vi "mclamp_set_holding.vi"(8 "error in (no error)":errorcluster, 9 "set holding (mV)":dbl, 10 "Error in":i32, 11 "Multiclamp Handle Out":u32) -> (0 "error out":errorcluster, 2 "error out":i32)   [LabVIEW 2015]
uses:
  multiBot/patcherBot/AxMultiClampMsg.dll
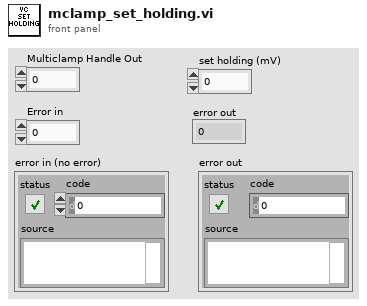
[diagram p1: front panel]
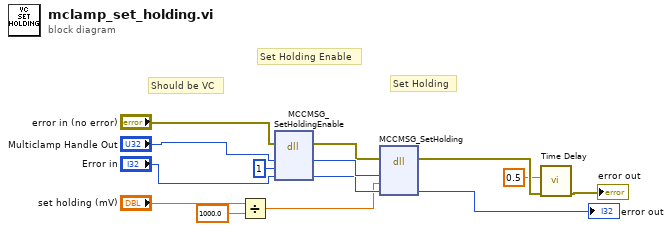
[diagram p0: block diagram]
diagram:
  # "Set Holding Enable"
  # "Set Holding"
  # "Should be VC"
  n1 = Divide(x="set holding (mV)", y=1000.0) -> (x/y=w3:dbl)
  n2 = dll-call lib="C:/multiBot/patcherBot/AxMultiClampMsg.dll" fn="MCCMSG_SetHoldingEnable"(error in="error in (no error)", "handle"="Multiclamp Handle Out", "ModeConstant"=1, "error"="Error in") -> (error out=w10:errorcluster, "handle"=w12:u32, "error"=w11:i32)  [unwired: 4 in, 1 out]
  n3 = dll-call lib="C:/multiBot/patcherBot/AxMultiClampMsg.dll" fn="MCCMSG_SetHolding"(error in=w10, "handle"=w12, "ModeConstant"=w3, "error"=w11) -> (error out=w6:errorcluster, "error"=→"error out":i32)  [unwired: 5 in, 1 out]
  n4 = call "Time Delay"("error in (no error)"=w6, "Delay Time (s)"=0.5) -> ("error out"=→"error out":errorcluster)  [unwired: 9 in]
